vi "Extract Planes.vi"(8 "error in (no error)":errorcluster, 11 "Images":T2) -> (0 "error out":errorcluster, 3 "Images":T2)   [LabVIEW 2015]
uses:
  controls/Images.ctl
  <vilib>/vision/Image Controls.llb/IMAQ Image.ctl
  <vilib>/vision/NI_Vision_Development_Module.lvlib
panel:
  out "Image Dst Out":T1(plugin-control)
  out "Image":T1(plugin-control)
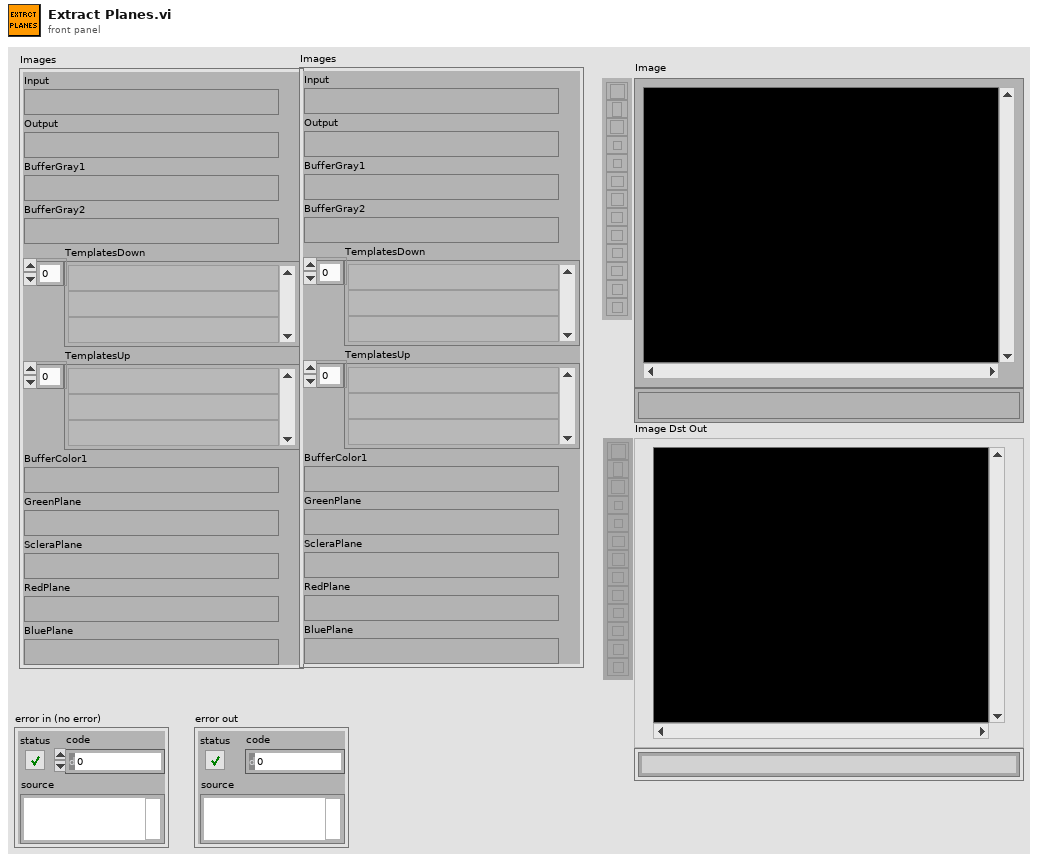
[diagram p1: front panel]
types:
  T1 = typedef "IMAQ Image.ctl" = refnum<image>
  T2 = typedef "Images.ctl" = cluster{"Input":T1, "Output":T1, "BufferGray1":T1, "BufferGray2":T1, "TemplatesDown":T1[], "TemplatesUp":T1[], "BufferColor1":T1, "GreenPlane":T1, "ScleraPlane":T1, "RedPlane":T1, "BluePlane":T1}
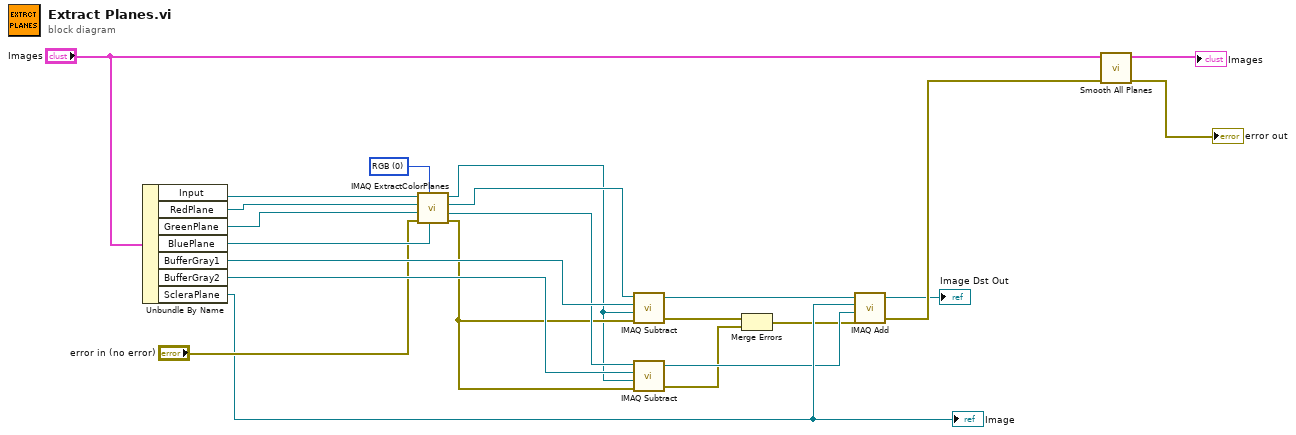
[diagram p0: block diagram]
diagram:
  w11 = u16 0 items=["RGB", "HSL", "HSV", "HSI"] ("Color Mode")
  n1 = Unbundle By Name("Images") -> ("Input"=w23:T1, "RedPlane"=w22:T1, "GreenPlane"=w21:T1, "BluePlane"=w20:T1, "BufferGray1"=w19:T1, "BufferGray2"=w18:T1, "ScleraPlane"=w16:T1)
  "Image" <- w16
  n2 = call "IMAQ ExtractColorPlanes"("Blue or Luma or Val or Inten Plane"=w20, "Color Mode"=w11, "error in (no error)"="error in (no error)", "Green or Sat Plane"=w21, "Red or Hue Plane"=w22, "Image Src"=w23) -> ("error out"=w7:errorcluster, "Blue or Luma or Val or Inten Plane out"=w10:T1, "Green or Sat Plane out"=w3:T1, "Red or Hue Plane out"=w2:T1)  [unwired: 2 in]
  n3 = call "IMAQ Subtract"("Image Src A"=w3, "Image Dst"=w19, "Image Src B"=w2, "error in (no error)"=w7) -> ("Image Dst Out"=w9:T1, "error out"=w6:errorcluster)  [unwired: 3 in]
  n4 = call "IMAQ Subtract"("Image Src A"=w10, "Image Dst"=w18, "Image Src B"=w2, "error in (no error)"=w7) -> ("Image Dst Out"=w8:T1, "error out"=w4:errorcluster)  [unwired: 3 in]
  n5 = Merge Errors(w6, w4) -> (w5:errorcluster)
  n6 = call "IMAQ Add"("Image Src A"=w9, "Image Dst"=w16, "Image Src B"=w8, "error in (no error)"=w5) -> ("Image Dst Out"=→"Image Dst Out":T1, "error out"=w13:errorcluster)  [unwired: 3 in]
  n7 = call "Smooth All Planes.vi"("error in (no error)"=w13, "Images"="Images") -> ("error out"=→"error out":errorcluster, "Images"=→"Images":T2)  [unwired: 8 in]
